vi "FTW-Connector-Connect.vi"(0 "FTW Actor Connector":refnum<class "FTW-Actor-Connector.lvclass">, 5 "Instance Inbox Address":string, 9 "Receive Message Size Limit":i32=1000000 format="%_4pbytes", 11 "error in":errorcluster) -> (4 "FTW Actor Connector out":refnum<class "FTW-Actor-Connector.lvclass">, 15 "error out":errorcluster)   [LabVIEW 2014, in "FTW-Actor-Connector.lvclass"]
doc: "Performs a \"cold call\" to connect to a running Actor Instance at the given Instance Inbox Address. Normally, this method is wrapped by a \"Construct\" method in each specific Actor Connector subclass."
uses:
  FTW-Actor-Connector.lvclass
  FTW-Actor-Connector.lvclass/FTW-Actor-Connector.ctl
panel:
  # "Inputs"
  # "Outputs"
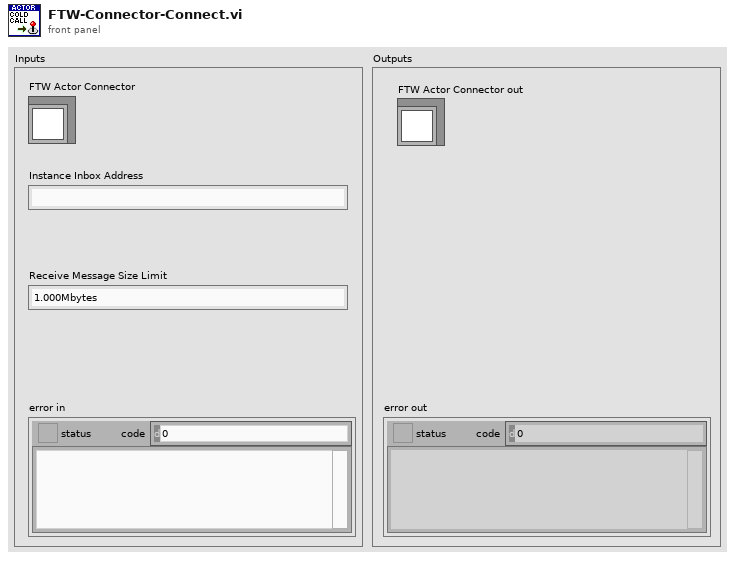
[diagram p1: front panel]
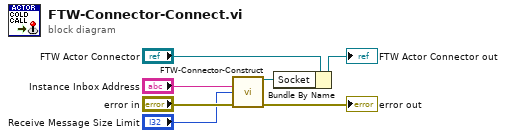
[diagram p0: block diagram]
diagram:
  n1 = call "FTW-Connector-Construct.vi"("Remote Inbox Address"="Instance Inbox Address", "Receive Message Size Limit"="Receive Message Size Limit", "error in"="error in") -> ("FTW Actor Connector"=w2:refnum<data-value>, "error out"=→"error out":errorcluster)  [unwired: 11 in]
  n2 = Bundle By Name(cluster="FTW Actor Connector", "Socket"=w2) -> (→"FTW Actor Connector out":refnum<class "FTW-Actor-Connector.lvclass">)
